vi "HSDIO_6541_Stop_Session.vi"(8 "error in (no error)":errorcluster, 11 "instrument handle in":refnum<k15>) -> (0 "error out":errorcluster)   [LabVIEW 2018]
doc: "I Description: FOR TESTS PURPOSE ONLY\nThis VI inits a waveform generation session for HSDIO 6541. This is a basic example that shows how to setup the board in order to generate waveforms according to a script. \n\nII Instructions for Running:\n1. Start the VI and select any previously created sequence script.\n2. If software trigger is choosen, just click on the Send Software Trigger button to generate the sequence.\nIf not, connect an external TTL trigger to the PFI0 input pin of the HSDIO, and generation will start immediately after the next trigger pulse.\n\nIII Block Diagram Steps:\n1. Initialize for a generation session.\n2. Assign the specified channels in Channel List for dynamic operation.\n3. Configure the Sample clock to use the onboard clock, and configure the clock rate.\n\n\n\n1. Initialize for a generation session.\n2. Assign specified channels in Channel List for dynamic operation : all = \"\" (default)\n3. Sets the Idle State for when the generation has completed : NO !!\n4. Configure the Sample clock to use the onboard clock, and configure the clock rate.\n5. Set generation mode to Scripted.\n6. Configure the Script Trigger : change to Digital Edge if waiting for an external\n trigger, and link Rising Edge and source trigger commands.\n Use PFI0 with SMB wired to the board, or any PFIxx if connected to accessory.\n6. Initiate dynamic pattern generation.\n7. Wait until the generation is done.\n8. Close the generation session."
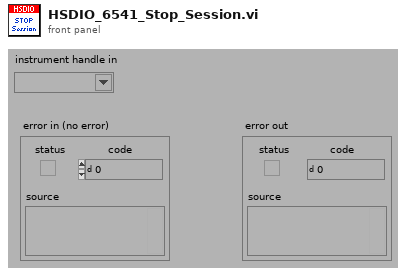
[diagram p1: front panel]
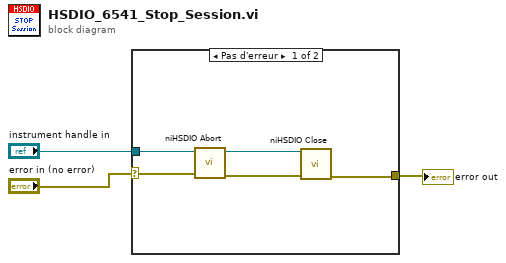
[diagram p0: block diagram]
diagram:
  n1 = case shown="Pas d'erreur" "error in (no error)" {
    selector: "error in (no error)" -> [w6 w9]
    tunnel: [w5 w9] -> w1
    tunnel: "instrument handle in" -> [w4 _]
    frame No Error {
      n2 = call <instrlib>:"niHSDIO Abort.vi"("error in (no error)"=w6, "instrument handle"=w4) -> ("error out"=w8:errorcluster, "instrument handle out"=w7:refnum<k15>)  [unwired: 8 in]
      n3 = call <instrlib>:"niHSDIO Close.vi"("error in (no error)"=w8, "instrument handle"=w7) -> ("error out"=w5:errorcluster)  [unwired: 9 in]
    }
    frame Error {
    }
  }
  "error out" <- w1
